vi "Light Open.vi"(7 "error in (no error)":errorcluster) -> (0 "error out":errorcluster, 3 "Lighting Refnum":refnum<k1>)   [LabVIEW 2018]
doc: "Opens the Theatre Lighting Hardware Device."
uses:
  Refnum Enum.ctl
panel:
  # "Input Data"
  # "Local Data"
  # "Output Data"
  # "No Local Data"
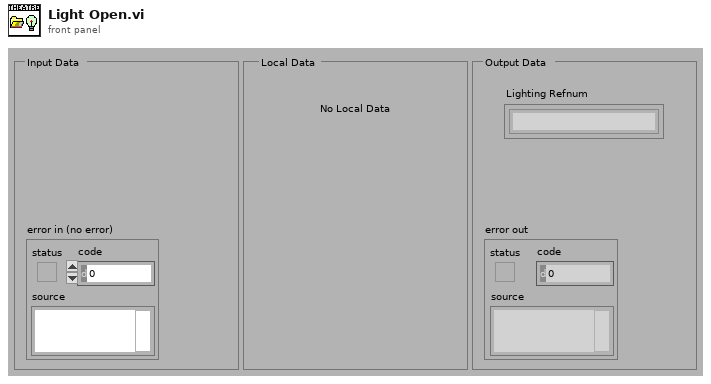
[diagram p1: front panel]
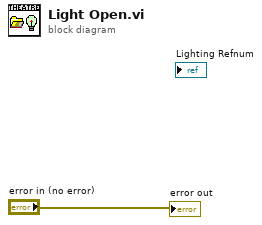
[diagram p0: block diagram]
diagram:
  "error out" <- "error in (no error)"
